vi "运维调试_氨氮.vi"() -> ()   [LabVIEW 2016, in "斯坦道氨氮.lvlib"]
uses:
  <vilib>/Utility/miscctls.llb/LVPointTypeDef.ctl
  <vilib>/Utility/config.llb/NI_LVConfig.lvlib
panel:
  in  "模块启用":bool
  in  "串口设置":bool
  in  "备用系数一键写入":bool
  in  "公式一键写入":bool
  in  "流程文件路径":path=path "C:/Users/Hsiao/Documents/斯坦道流程文件/流程.xml"
  in  "曲线模型":cluster{"X^2":dbl, "X":dbl, "B":dbl}(xcontrol)
  in  "质控参数设置":bool
  out "字符串":string
  in  "氨氮自动测试量程配置":T1
  out "ADC":sgl
  out "温度2":sgl
  out "温度1":sgl
  out "固件版本号":string
  in  "数组":string[](array[string])
  in  "备用系数写入":bool
  in  "备用系数读取":bool
  in  "备用系数":T2
  in  "量程切换阈值写入":bool
  in  "量程切换阈值读取":bool
  in  "量程切换阈值":cluster{"阈值":dbl, "标液浓度":dbl}
  in  "参数下拉列表":enum16{"氨氮", "总磷"}(ring)
  in  "量程下拉列表":enum16{"低量程", "高量程"}(ring)
  in  "测量模式下拉列表":enum16{"水样测量", "空白核查", "跨度核查", "标样核查", "加标回收"}(ring)
  in  "公式":cluster{"X^2":dbl, "X":dbl, "b":dbl}
  in  "写公式":bool
  in  "读公式":bool
  in  "返回":bool
  in  "设置":bool
  out "序列号":string="序列号"
  out "氨氮测量数据":T3(xcontrol)
  out "集成报警信息":string
  out "定时启动":bool
  out "总磷总氮运行状态":T4(xcontrol)
  in  "停止":bool
  in  "手动启动":bool
  in  "单步测试":bool
  in  "总磷氨氮调试":u16[](xcontrol)
  out "F3":sgl format="%#.6f"
  out "F2":sgl format="%#.6f"
  out "F1":sgl format="%#.6f"
  out "F0":sgl format="%#.6f"
  out "多列列表框":i32(listbox)
  # "参数设置"
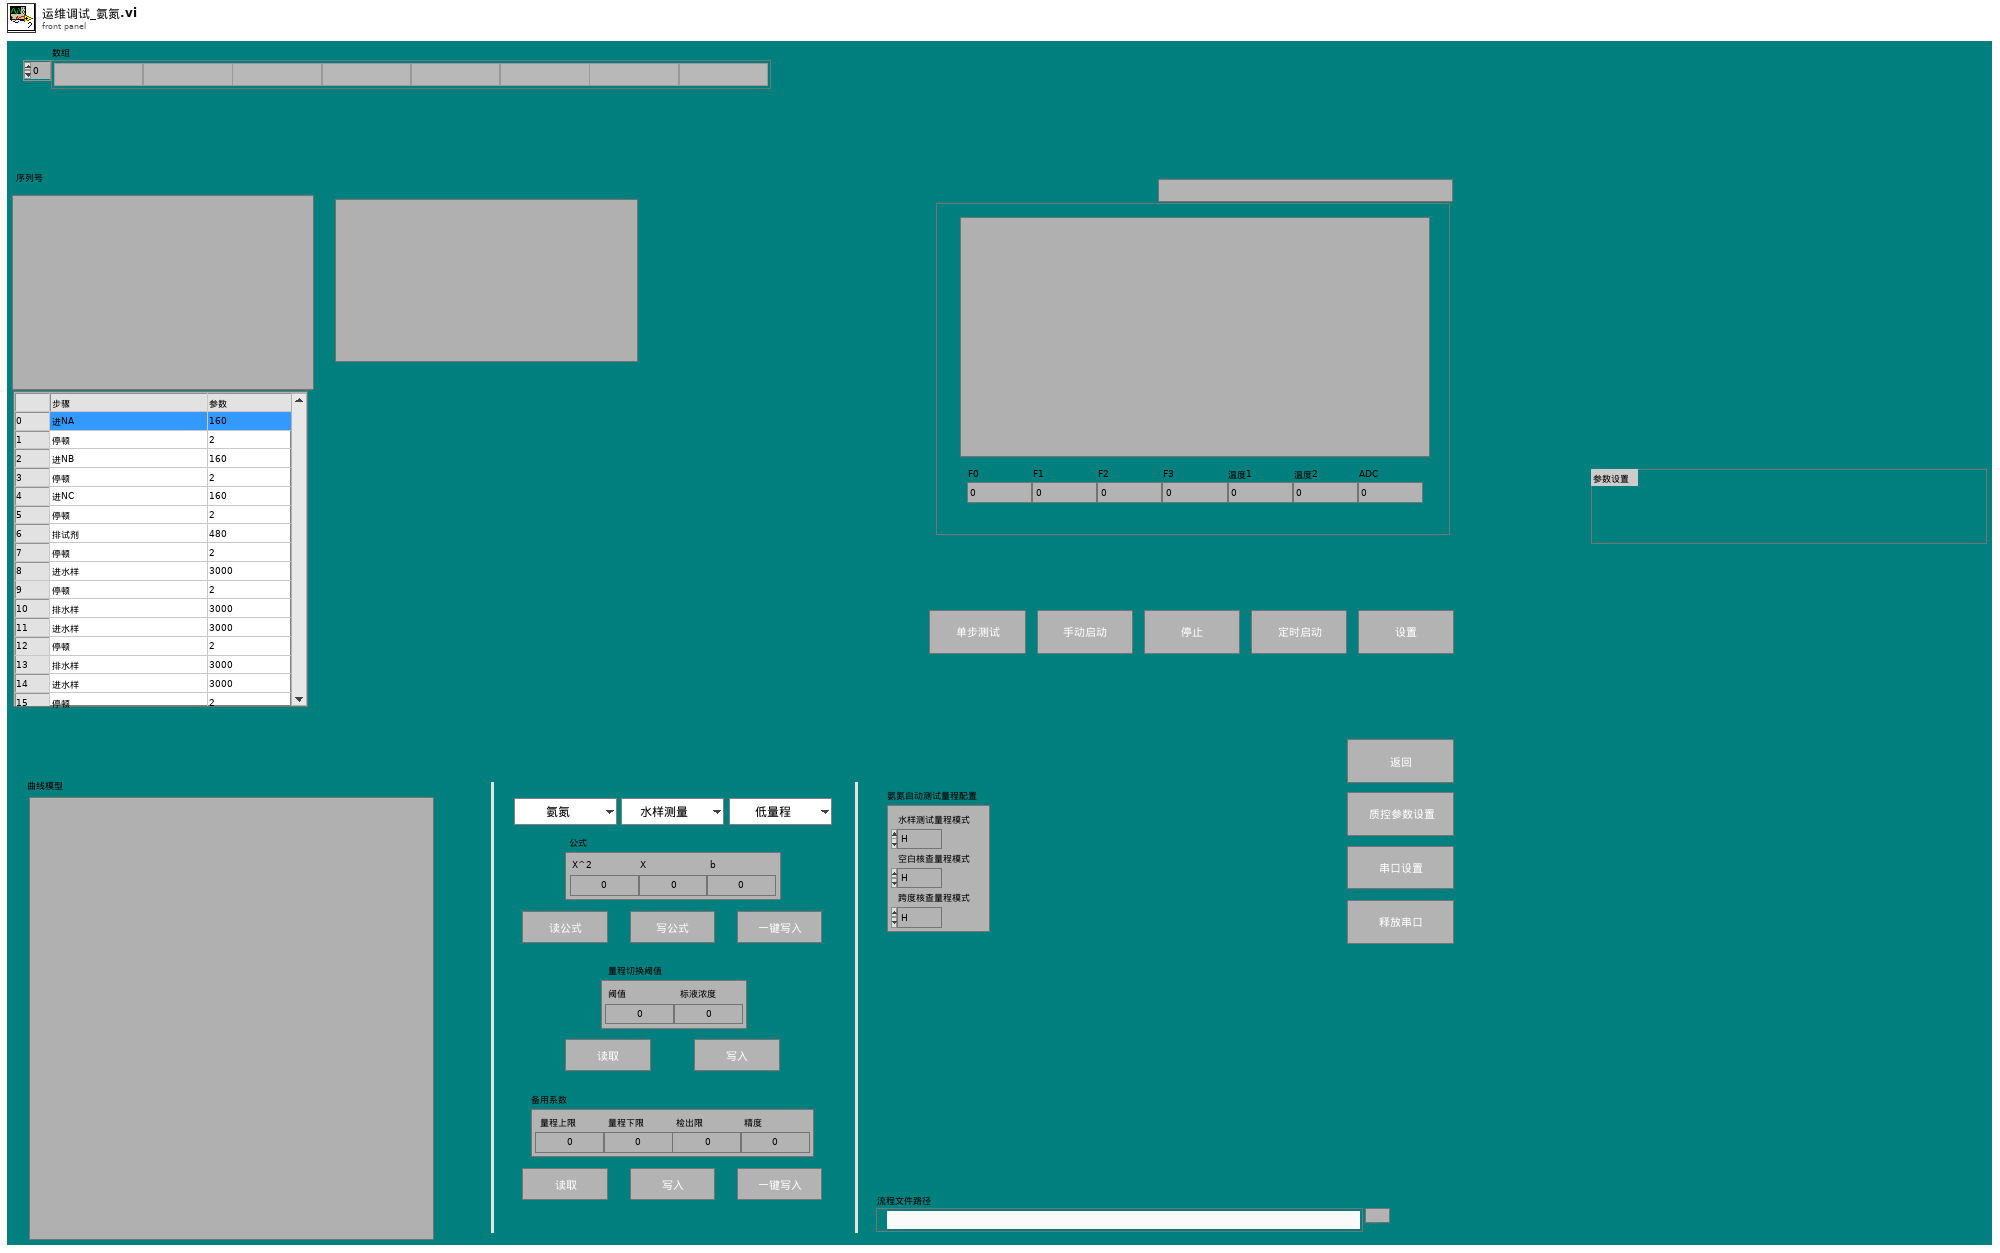
[diagram p1: front panel]
types:
  T1 = cluster{"水样测试量程模式":enum16{"H", "L", "AUTO"}, "空白核查量程模式":enum16{"H", "L", "AUTO"}, "跨度核查量程模式":enum16{"H", "L", "AUTO"}}
  T2 = cluster{"量程上限":dbl, "量程下限":dbl, "检出限":dbl, "精度":dbl}
  T3 = cluster{"flowid":u16, "测量精度":u16, "测量数据区":cluster{"因子编码":u32, "单位":u16, "标样参考值":sgl, "水样数据时间":timestamp, "水样实测值":sgl, "水样数据标识":string, "标样数据时间":timestamp, "标样实测值":sgl, "标样数据标识":string, "空白数据时间":timestamp, "空白实测值":sgl, "空白数据标识":string, "零点核查数据时间":timestamp, "零点核查实测值":sgl, "零点核查数据标识":string, "跨度核查数据时间":timestamp, "跨度核查实测值":sgl, "跨度核查数据标识":string, "加标回收数据时间":timestamp, "加标回收实测值":sgl, "加标回收数据标识":string, "平行样数据时间":timestamp, "平行样实测值":sgl, "平行样数据标识":string}}
  T4 = cluster{"系统时间":timestamp, "工作状态":enum16{"空闲", "水样测试", "标样核查", "零点核查", "跨度核查", "空白测试", "平行样测试", "加标回收", "空白校准", "标样校准", "初始化（清洗）"}, "测量模式":enum16{"待机", "连续模式", "周期模式", "定点模式", "受控模式", "手动模式"}, "告警代码":enum16{"无告警", "缺试剂告警", "缺水样告警", "缺蒸馏水告警", "缺标液告警", "仪表漏液告警", "标定异常告警", "超量程告警", "加热异常", "低试剂预警", "超上限告警", "超下限告警", "仪表内部其他异常", "滴定异常告警", "电极异常告警", "量程切换告警", "参数设置告警", "PH电极电位异常", "电导率电极异常", "浊度光度异常", "溶解氧电极异常", "溶解氧光强异常", "温度异常告警", "PH异常告警", "溶解氧异常告警", "电导率异常告警", "浊度异常告警", "叶绿素异常告警", "藻密度异常告警", "蓝绿藻异常告警", "ORP异常告警", "氨氮异常告警", "清洁刷异常告警", "SD卡异常告警", "蓝牙异常告警", "Wifi异常告警", "流程异常告警"}, "故障代码":enum16{"无故障", "电机故障", "温度故障", "通讯故障", "滴定故障"}, "日志代码":u16, "软件版本":u16, "F0":sgl, "F1":sgl, "F2":sgl, "F3":sgl, "T":sgl, "H":sgl, "id":u16, "flowid":u16, "量程":u16, "总磷控温温度1":sgl, "营养盐控温温度2":sgl, "ADC":sgl}
  T5 = cluster{"站号":u16, "量程切换":enum32{"H", "L", "AUTO"}, "控制命令":enum16{"启动测量", "标样核查", "零点核查", "跨度核查", "空白测试", "平行样测试", "加标回收", "空白校准", "标样校准", "初始化（清洗）", "停止测试", "仪器重启", "校时", "模式设置", "测量间隔设置"}, "模式设置":enum16{"待机", "连续模式", "周期模式", "定点模式", "受控模式", "手动模式"}, "测量间隔":u16}
  T6 = enum16{"启动测量", "标样核查", "零点核查", "跨度核查", "空白测试", "平行样测试", "加标回收", "空白校准", "标样校准", "初始化（清洗）", "停止测试", "仪器重启", "校时", "模式设置", "测量间隔设置"}
  T7 = cluster{"仪器测试类型":enum16{"水样测试", "标样核查", "空白测试", "跨度核查"}, "周期设置类型":enum16{"定点启动", "间隔启动"}, "定时功能启用":bool, "定时间隔":dbl, "24H周期设置":bool[]}
  T8 = enum32{"Bad", "Idle", "Run top level", "Running"}
  T9 = typedef "LVDateTimeRec.ctl" = cluster{"秒数的小数部分":dbl, "秒":i32, "分":i32, "时":i32, "日":i32, "月":i32, "年":i32, "天数（周）":i32, "天数（年）":i32, "DST":i32}
  T10 = typedef "LVPointTypeDef.ctl" = cluster{"Horizontal":i16, "Vertical":i16}
  T11 = cluster{"因子编码":u32, "单位":u16, "标样参考值":sgl, "水样数据时间":timestamp, "水样实测值":sgl, "水样数据标识":string, "标样数据时间":timestamp, "标样实测值":sgl, "标样数据标识":string, "空白数据时间":timestamp, "空白实测值":sgl, "空白数据标识":string, "零点核查数据时间":timestamp, "零点核查实测值":sgl, "零点核查数据标识":string, "跨度核查数据时间":timestamp, "跨度核查实测值":sgl, "跨度核查数据标识":string, "加标回收数据时间":timestamp, "加标回收实测值":sgl, "加标回收数据标识":string, "平行样数据时间":timestamp, "平行样实测值":sgl, "平行样数据标识":string}
  T12 = enum16{"空闲", "水样测试", "标样核查", "零点核查", "跨度核查", "空白测试", "平行样测试", "加标回收", "空白校准", "标样校准", "初始化（清洗）"}
  T13 = cluster{"启动模式":enum16{"跨度核查", "水样测量", "空白核查", "标样核查", "加标回收"}, "启动参数":u16, "量程":enum16{"低量程", "高量程"}}
  T14 = cluster{"时间标识":timestamp, "设备":string, "日志信息":string, "流程参数":string}
  T15 = cluster{"时间标识":timestamp, "设备":string, "日志信息":string}
  T16 = enum16{"无告警", "缺试剂告警", "缺水样告警", "缺蒸馏水告警", "缺标液告警", "仪表漏液告警", "标定异常告警", "超量程告警", "加热异常", "低试剂预警", "超上限告警", "超下限告警", "仪表内部其他异常", "滴定异常告警", "电极异常告警", "量程切换告警", "参数设置告警", "PH电极电位异常", "电导率电极异常", "浊度光度异常", "溶解氧电极异常", "溶解氧光强异常", "温度异常告警", "PH异常告警", "溶解氧异常告警", "电导率异常告警", "浊度异常告警", "叶绿素异常告警", "藻密度异常告警", "蓝绿藻异常告警", "ORP异常告警", "氨氮异常告警", "清洁刷异常告警", "SD卡异常告警", "蓝牙异常告警", "Wifi异常告警", "流程异常告警"}
  T17 = typedef "LVRowAndColumnUnsignedTypeDef.ctl" = cluster{"Row":u32, "Column":u32}
  T18 = typedef "NI_LVConfig.lvlib/Config Data RefNum.ctl" = refnum<k1>
  T19 = cluster{"跨度值":dbl, "零点标准液浓度":dbl, "跨度标准液浓度":dbl, "标准液标准浓度":dbl}
  T20 = cluster{"确定":bool, "跨度值":dbl, "零点标准液浓度":dbl, "跨度标准液浓度":dbl, "标准液标准浓度":dbl}
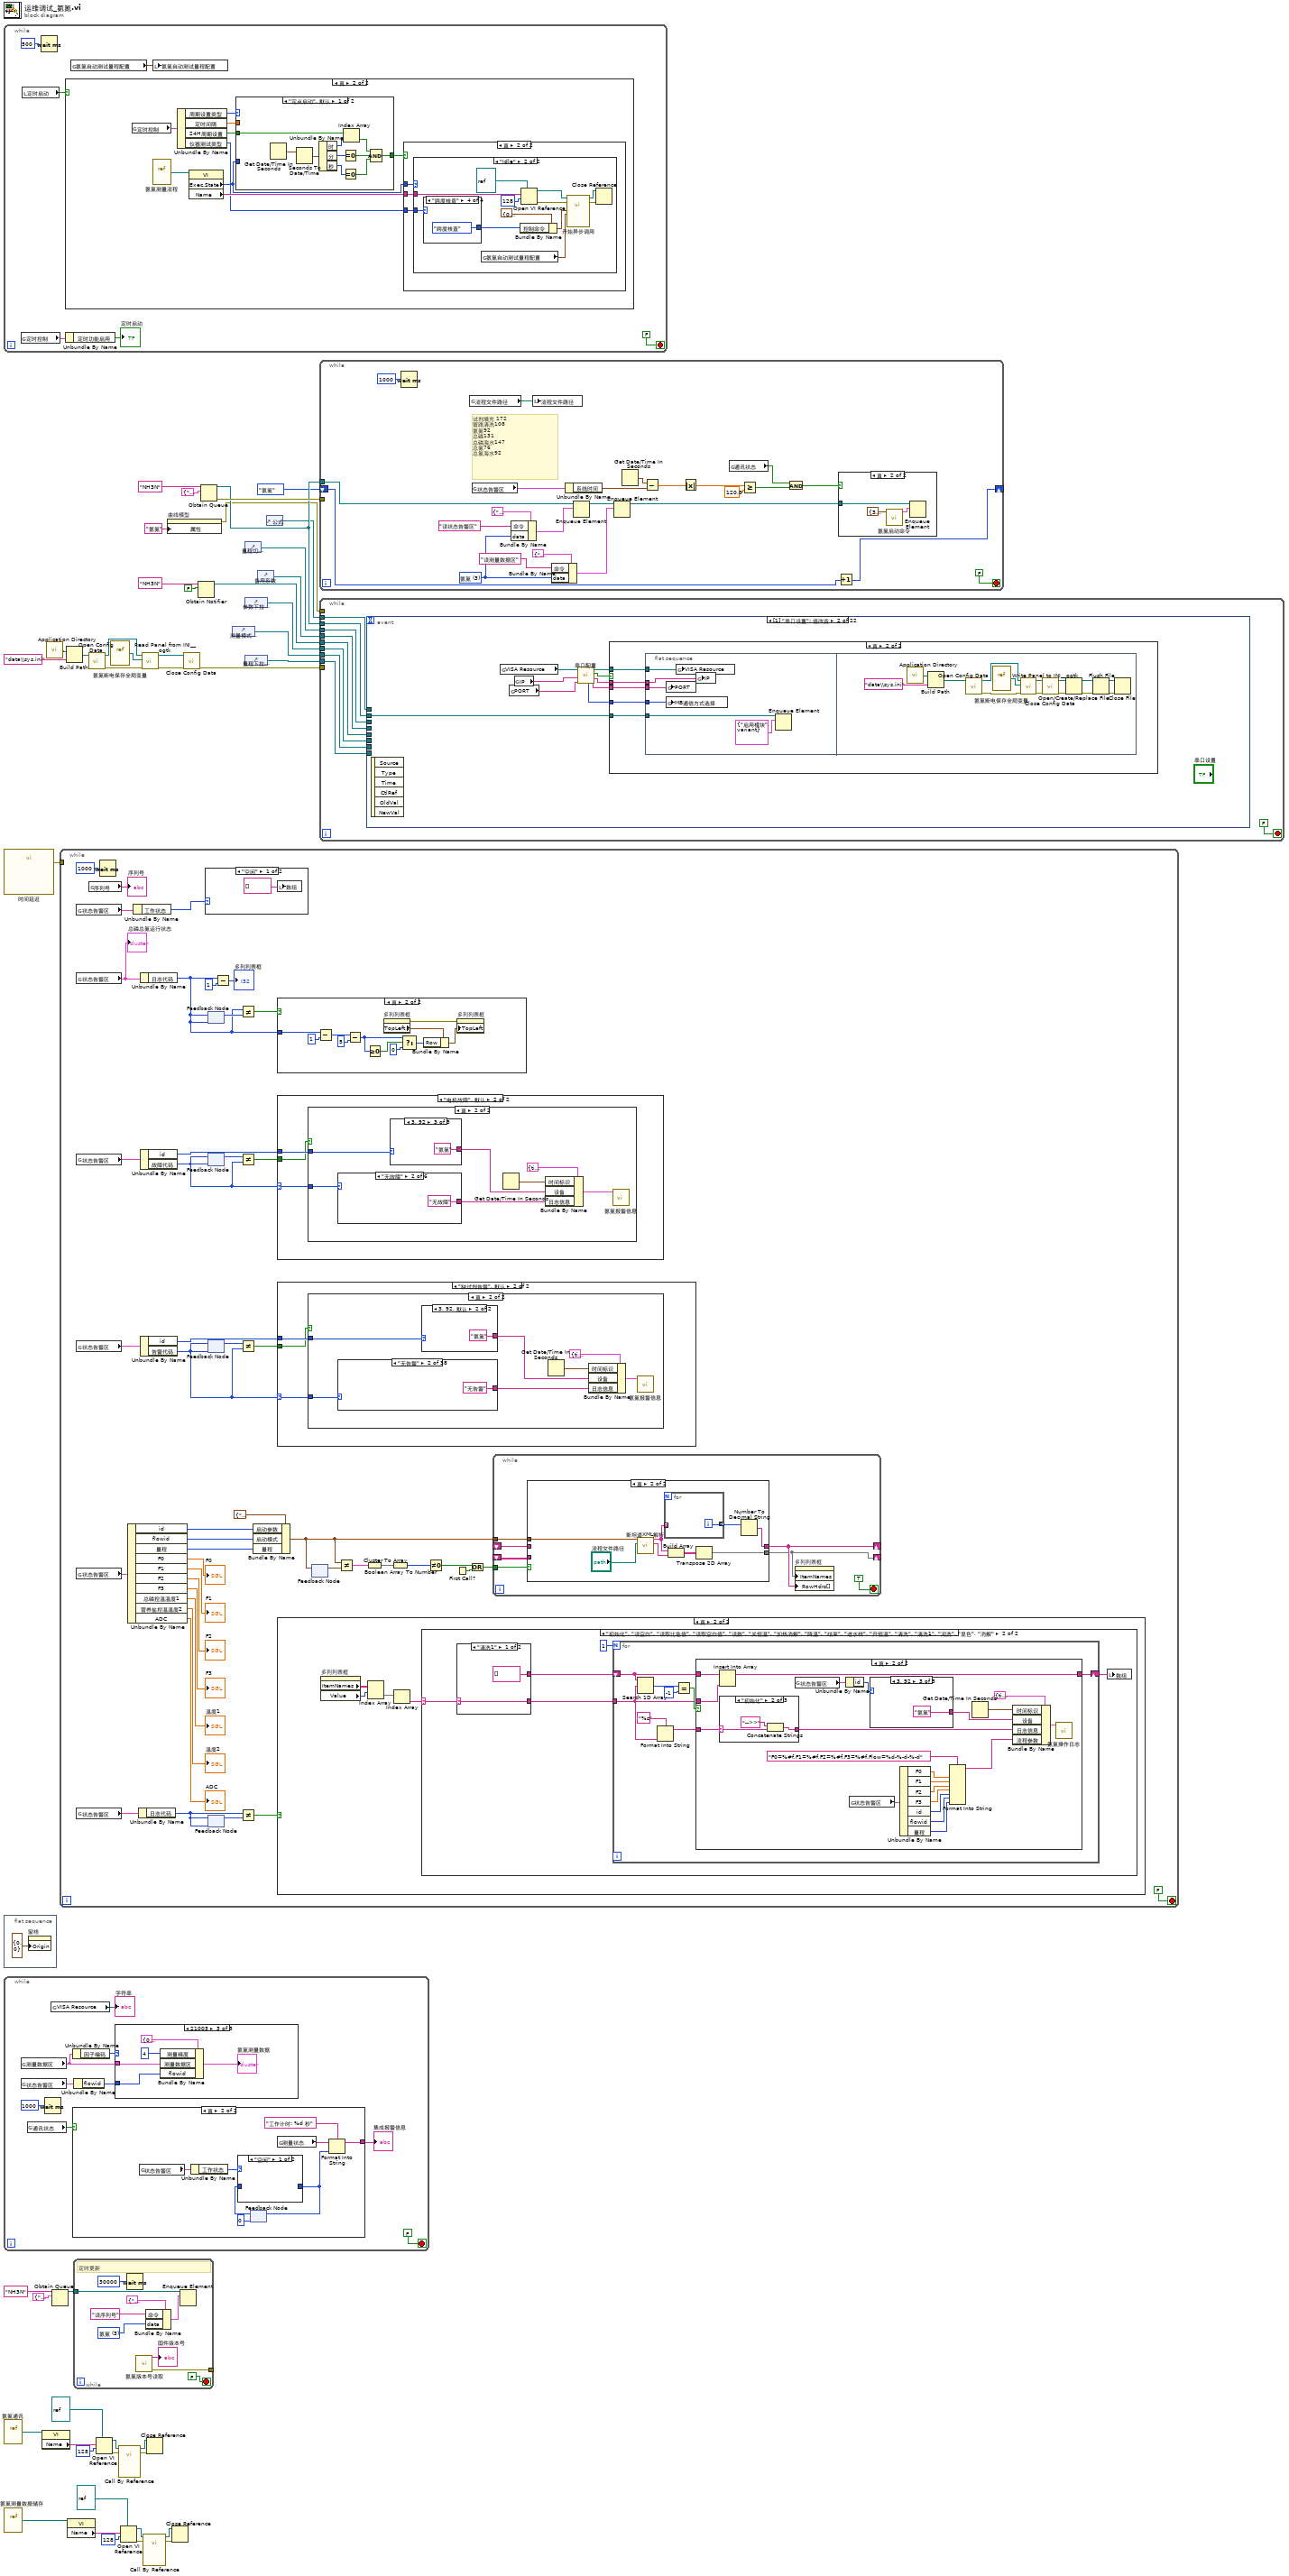
[diagram p0: block diagram]
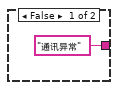
[diagram p2: hidden frame]
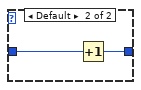
[diagram p3: hidden frame]
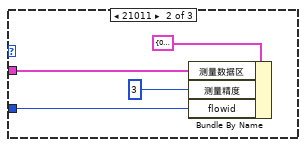
[diagram p5: hidden frame]
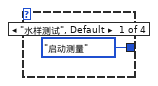
[diagram p9: hidden frame]
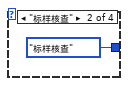
[diagram p10: hidden frame]
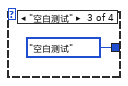
[diagram p11: hidden frame]
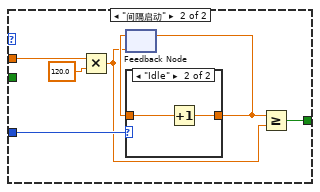
[diagram p12: hidden frame]
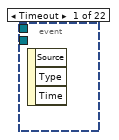
[diagram p14: hidden frame]
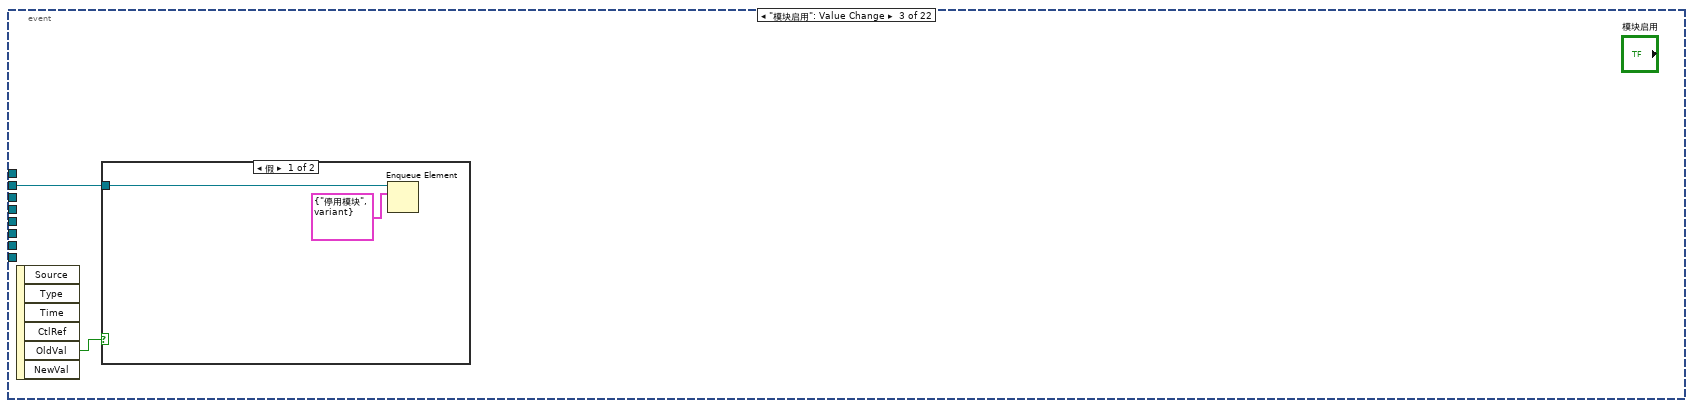
[diagram p16: hidden frame]
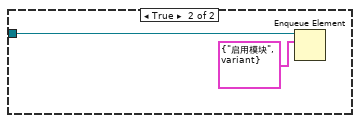
[diagram p17: hidden frame]
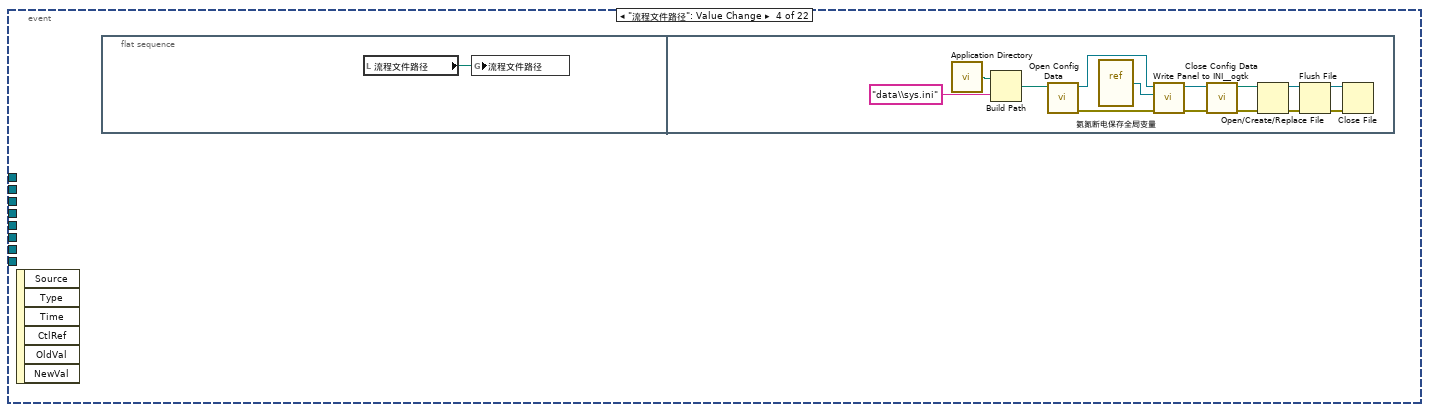
[diagram p18: hidden frame]
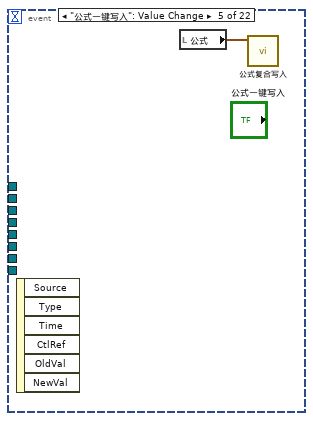
[diagram p19: hidden frame]
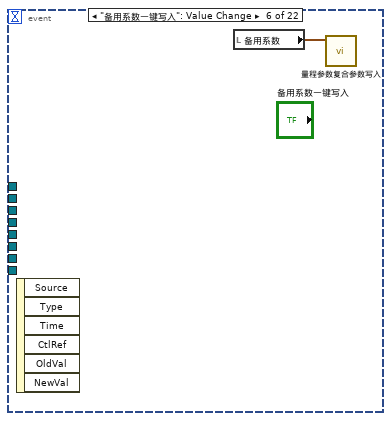
[diagram p20: hidden frame]
diagram:
  n1 = while {
    stop <- FALSE stop-if-true
    n2 = global read "氨氮断电保存全局变量.vi" "定时控制"() -> (w48:T7)
    n3 = local read "定时启动"() -> (w49:bool)
    n4 = Wait (ms)(milliseconds to wait=u32 500 ("等待时间（毫秒）")) -> ()  [unwired: 1 out]
    n5 = case shown="真" w49 {
      frame False {
      }
      frame True {
        n6 = global read "氨氮断电保存全局变量.vi" "定时控制"() -> (w60:T7)
        n7 = vi-ref "氨氮测量流程.vi"() -> (w56:refnum<vi>)
        n8 = Unbundle By Name(w60) -> ("周期设置类型"=w59:enum16{"定点启动", "间隔启动"}, "定时间隔"=w58:dbl, "24H周期设置"=w57:bool[], "仪器测试类型"=w53:enum16{"水样测试", "标样核查", "空白测试", "跨度核查"})
        n9 = property class="VI"(reference=w56) -> ("Exec.State"=w52:T8, "Name"=w55:string)  [unwired: 1 in, 2 out]
        n10 = case shown="\"定点启动\", 默认" w59 {
          tunnel: w58 -> [_ w93]
          tunnel: w57 -> [w89 _]
          tunnel: w52 -> [_ w96]
          tunnel: [w88 w91] -> w54
          frame "定点启动", Default {
            n11 = Get Date/Time In Seconds() -> (seconds since 1Jan1904=w87:timestamp)
            n12 = Seconds To Date/Time(time stamp (now)=w87) -> (date time rec=w86:T9)  [unwired: 1 in]
            n13 = Unbundle By Name(w86) -> ("时"=w85:i32, "分"=w83:i32, "秒"=w84:i32)
            n14 = Equal To 0?(x=w83) -> (x = 0?=w81:bool)
            n15 = Equal To 0?(x=w84) -> (x = 0?=w80:bool)
            n16 = Index Array(array=w89, index=w85) -> (element=w82:bool)
            n17 = Compound Arithmetic op=AND ("复合运算")(w82, w81, w80) -> (w88:bool)
          }
          frame "间隔启动" {
            n18 = Multiply(x=w93, y=120.0) -> (x*y=w90:dbl)
            n19 = feedback #1(w90) -> (w95:dbl)
            n20 = case shown="\"Idle\"" w96 {
              tunnel: w95 -> [_ w98]
              tunnel: [_ w97] -> w94
              frame "Bad", Default {
              }
              frame "Idle" {
                n21 = Increment(x=w98) -> (x+1=w97:dbl)
              }
            }
            n22 = feedback-in #1(w94) -> ()
            n23 = Greater Or Equal?(x=w94, y=w90) -> (x >= y?=w91:bool)
          }
        }
        n24 = case shown="真" w54 {
          tunnel: w55 -> [_ w63]
          tunnel: w53 -> [_ w62]
          tunnel: w52 -> [_ w61]
          frame False {
          }
          frame True {
            n25 = case shown="\"Idle\"" w61 {
              tunnel: w63 -> [_ w70]
              tunnel: w62 -> [_ w66]
              frame "Bad", Default {
              }
              frame "Idle" {
                n26 = case shown="\"跨度核查\"" w66 {
                  tunnel: [T6."启动测量" ("控制命令") T6."标样核查" ("控制命令") T6."空白测试" ("控制命令") T6."跨度核查" ("控制命令")] -> w65
                  frame "水样测试", Default {
                  }
                  frame "标样核查" {
                  }
                  frame "空白测试" {
                  }
                  frame "跨度核查" {
                  }
                }
                n27 = global read "氨氮断电保存全局变量.vi" "氨氮自动测试量程配置"() -> (w64:T1)
                n28 = Bundle By Name(cluster=T5 {"站号"=0, "量程切换"=enum."H", "控制命令"=enum."启动测量", "模式设置"=enum."待机", "测量间隔"=0} ("参数"), "控制命令"=w65) -> (w67:T5)
                n29 = Open VI Reference(type specifier VI Refnum (for type only)=refnum<vi> refnum, vi path=w70, options=128 ("选项")) -> (vi reference=w71:refnum<vi>, error out=w72:errorcluster)  [unwired: 3 in]
                n30 = call-by-ref "开始异步调用"(reference=w71, error in=w72, "量程模式"=w64, "参数"=w67) -> (reference out=w73:refnum<vi>, error out=w74:errorcluster)  [unwired: 10 in]
                n31 = Close Reference(reference=w73, error in (no error)=w74) -> ()  [unwired: 1 out]
              }
            }
          }
        }
      }
    }
    n32 = Unbundle By Name(w48) -> ("定时功能启用"=→"定时启动":bool)
    n33 = global read "氨氮断电保存全局变量.vi" "氨氮自动测试量程配置"() -> (w46:T1)
    n34 = local write "氨氮自动测试量程配置"(w46) -> ()
  }
  n35 = call "时间延迟"() -> ("error out"=w18:errorcluster)  [unwired: 11 in]
  n36 = flat-sequence {
    frame #0 {
      n37 = property on="窗格" class="Pane"("Origin"=T10 {"Horizontal"=0, "Vertical"=0} ("原点")) -> ()  [unwired: 2 in, 2 out]
    }
  }
  n38 = while {
    stop <- FALSE stop-if-true
    n39 = global read "VAR氨氮全局变量.vi" "测量数据区"() -> (w106:T11)
    n40 = global read "VAR氨氮全局变量.vi" "状态告警区"() -> (w102:T4)
    n41 = global read "VAR氨氮全局变量.vi" "通讯状态"() -> (w104:bool)
    n42 = Wait (ms)(milliseconds to wait=u32 1000 ("等待时间（毫秒）")) -> ()  [unwired: 1 out]
    n43 = global read "氨氮断电保存全局变量.vi" "VISA Resource"() -> (→"字符串":refnum<visa-resource-name>)
    n44 = Unbundle By Name(w106) -> ("因子编码"=w105:u32)
    n45 = case shown="真" w104 {
      tunnel: ["通讯异常" ("集成报警信息") w111] -> w103
      frame False {
      }
      frame True {
        n46 = global read "VAR氨氮全局变量.vi" "状态告警区"() -> (w117:T4)
        n47 = Unbundle By Name(w117) -> ("工作状态"=w116:T12)
        n48 = feedback #2(0) -> (w114:i32)
        n49 = case shown="\"空闲\"" w116 {
          tunnel: w114 -> [_ w119]
          tunnel: [_ w118] -> w112
          frame "空闲" {
          }
          frame Default {
            n50 = Increment(x=w119) -> (x+1=w118:i32)
          }
        }
        n51 = feedback-in #2(w112) -> ()
        n52 = global read "VAR氨氮全局变量.vi" "测量状态"() -> (w110:string)
        n53 = Format Into String(format string="工作计时: %d 秒" ("格式字符串"), initial string=w110, w112) -> (resulting string=w111:string)  [unwired: 1 in, 1 out]
      }
    }
    "集成报警信息" <- w103
    n54 = Unbundle By Name(w102) -> ("flowid"=w101:u16)
    n55 = case shown="21003" w105 {
      tunnel: w106 -> [_ w123 w128]
      tunnel: w101 -> [_ w121 w126]
      frame Default {
      }
      frame 21011 {
        n56 = Bundle By Name(cluster=T3 {"flowid"=0, "测量精度"=0, "测量数据区"={"因子编码"=0, "单位"=0, "标样参考值"=0.0, "水样数据时间"=timestamp(0 s since 1904-01-01), "水样实测值"=0.0, "水样数据标识"="", "标样数据时间"=timestamp(0 s since 1904-01-01), "标样实测值"=0.0, "标样数据标识"="", "空白数据时间"=timestamp(0 s since 1904-01-01), "空白实测值"=0.0, "空白数据标识"="", "零点核查数据时间"=timestamp(0 s since 1904-01-01), "零点核查实测值"=0.0, "零点核查数据标识"="", "跨度核查数据时间"=timestamp(0 s since 1904-01-01), "跨度核查实测值"=0.0, "跨度核查数据标识"="", "加标回收数据时间"=timestamp(0 s since 1904-01-01), "加标回收实测值"=0.0, "加标回收数据标识"="", "平行样数据时间"=timestamp(0 s since 1904-01-01), "平行样实测值"=0.0, "平行样数据标识"=""}} ("氨氮测量数据"), "测量数据区"=w123, "测量精度"=u16 3, "flowid"=w121) -> ()  [unwired: 1 out]
      }
      frame 21003 {
        n57 = Bundle By Name(cluster=T3 {"flowid"=0, "测量精度"=0, "测量数据区"={"因子编码"=0, "单位"=0, "标样参考值"=0.0, "水样数据时间"=timestamp(0 s since 1904-01-01), "水样实测值"=0.0, "水样数据标识"="", "标样数据时间"=timestamp(0 s since 1904-01-01), "标样实测值"=0.0, "标样数据标识"="", "空白数据时间"=timestamp(0 s since 1904-01-01), "空白实测值"=0.0, "空白数据标识"="", "零点核查数据时间"=timestamp(0 s since 1904-01-01), "零点核查实测值"=0.0, "零点核查数据标识"="", "跨度核查数据时间"=timestamp(0 s since 1904-01-01), "跨度核查实测值"=0.0, "跨度核查数据标识"="", "加标回收数据时间"=timestamp(0 s since 1904-01-01), "加标回收实测值"=0.0, "加标回收数据标识"="", "平行样数据时间"=timestamp(0 s since 1904-01-01), "平行样实测值"=0.0, "平行样数据标识"=""}} ("氨氮测量数据"), "测量精度"=u16 4, "测量数据区"=w128, "flowid"=w126) -> (→"氨氮测量数据":T3)
      }
    }
  }
  n58 = vi-ref "氨氮通讯.vi"() -> (w41:refnum<vi>)
  n59 = vi-ref "氨氮测量数据储存.vi"() -> (w33:refnum<vi>)
  n60 = property class="VI"(reference=w41) -> ("Name"=w40:string)  [unwired: 1 in, 2 out]
  n61 = call <vilib>:"Application Directory.vi"() -> ("Application Directory"=w4:path)
  n62 = Obtain Queue(name (unnamed)="NH3N" ("名称（未命名）"), element data type=cluster{"命令":string, "data":variant} {"命令"="", "data"=variant}) -> (queue out=w15:refnum<queue>)  [unwired: 3 in, 2 out]
  n63 = while {
    tunnel: w18 -> [_]
    stop <- FALSE stop-if-true
    n64 = global read "VAR氨氮全局变量.vi" "状态告警区"() -> (w141:T4)
    n65 = global read "VAR氨氮全局变量.vi" "状态告警区"() -> (w154:T4)
    "总磷总氮运行状态" <- w154
    n66 = global read "VAR氨氮全局变量.vi" "状态告警区"() -> (w146:T4)
    n67 = global read "VAR氨氮全局变量.vi" "状态告警区"() -> (w151:T4)
    n68 = global read "VAR氨氮全局变量.vi" "状态告警区"() -> (w162:T4)
    n69 = global read "VAR氨氮全局变量.vi" "状态告警区"() -> (w138:T4)
    n70 = global read "VAR氨氮全局变量.vi" "序列号"() -> (→"序列号":string)
    n71 = Wait (ms)(milliseconds to wait=u32 1000 ("等待时间（毫秒）")) -> ()  [unwired: 1 out]
    n72 = Unbundle By Name(w162) -> ("id"=w159:u16, "flowid"=w161:u16, "量程"=w160:u16, "F0"=→"F0":sgl, "F1"=→"F1":sgl, "F2"=→"F2":sgl, "F3"=→"F3":sgl, "总磷控温温度1"=→"温度1":sgl, "营养盐控温温度2"=→"温度2":sgl, "ADC"=→"ADC":sgl)
    n73 = Unbundle By Name(w141) -> ("工作状态"=w140:T12)
    n74 = Unbundle By Name(w138) -> ("日志代码"=w137:u16)
    n75 = Unbundle By Name(w154) -> ("日志代码"=w131:u16)
    n76 = Unbundle By Name(w146) -> ("id"=w145:u16, "故障代码"=w142:enum16{"无故障", "电机故障", "温度故障", "通讯故障", "滴定故障"})
    n77 = Unbundle By Name(w151) -> ("id"=w150:u16, "告警代码"=w147:T16)
    n78 = case shown="\"空闲\"" w140 {
      frame "空闲" {
        n79 = local write "数组"(string[] [] ("数组")) -> ()
      }
      frame "水样测试", Default {
      }
    }
    n80 = feedback-in #3(w131) -> ()
    n81 = feedback #3(w131) -> (w171:u16)
    n82 = feedback #4(w142) -> (w143:enum16{"无故障", "电机故障", "温度故障", "通讯故障", "滴定故障"})
    n83 = feedback-in #4(w142) -> ()
    n84 = feedback #5(w147) -> (w148:T16)
    n85 = feedback-in #5(w147) -> ()
    n86 = feedback #6(w137) -> (w139:u16)
    n87 = feedback-in #6(w137) -> ()
    n88 = Subtract(x=w131, y=1) -> (x-y=→"多列列表框":i32)
    n89 = Not Equal?(x=w131, y=w171) -> (x != y?=w170:bool)
    n90 = Not Equal?(x=w143, y=w142) -> (x != y?=w144:bool)
    n91 = Not Equal?(x=w148, y=w147) -> (x != y?=w149:bool)
    n92 = Not Equal?(x=w137, y=w139) -> (x != y?=w136:bool)
    n93 = Bundle By Name(cluster=T13 {"启动模式"=enum."跨度核查", "启动参数"=1, "量程"=enum."低量程"} ("参数簇"), "启动参数"=w159, "启动模式"=w161, "量程"=w160) -> (w153:T13)
    n94 = case shown="真" w170 {
      tunnel: w131 -> [_ w321]
      frame False {
      }
      frame True {
        n95 = Subtract(x=w321, y=1) -> (x-y=w319:i32)
        n96 = Subtract(x=w319, y=5) -> (x-y=w323:i32)
        n97 = Greater Or Equal To 0?(x=w323) -> (x >= 0?=w322:bool)
        n98 = property on="多列列表框" class="MCListbox (严格)"() -> (error out=w327:errorcluster, "TopLeft"=w328:T17)  [unwired: 2 in, 1 out]
        n99 = Select(t=w323, s=w322, f=0) -> (s? t:f=w324:i32)
        n100 = Bundle By Name(cluster=w328, "Row"=w324) -> (w329:T17)
        n101 = property on="多列列表框" class="MCListbox (严格)"(error in=w327, "TopLeft"=w329) -> ()  [unwired: 1 in, 2 out]
      }
    }
    n102 = case shown="\"电机故障\", 默认" w142 {
      selector: w142 -> [_ w228]
      tunnel: w145 -> [_ w229]
      tunnel: w144 -> [_ w227]
      frame "无故障" {
      }
      frame "电机故障", Default {
        n103 = case shown="真" w227 {
          tunnel: w229 -> [_ w236]
          tunnel: w228 -> [_ w231]
          frame False {
          }
          frame True {
            n104 = case shown="\"无故障\"" w231 {
              selector: w231 -> [w238 _ _ _ _ _]
              tunnel: [w237 "无故障" "电机故障" "温度故障" "通讯故障" "滴定故障"] -> w230
              frame Default {
                n105 = Format Into String(format string="%d" ("格式字符串"), initial string="未知" ("工作状态"), w238) -> (resulting string=w237:string)  [unwired: 1 in, 1 out]
              }
              frame "无故障" {
              }
              frame "电机故障" {
              }
              frame "温度故障" {
              }
              frame "通讯故障" {
              }
              frame "滴定故障" {
              }
            }
            n106 = case shown="3, 92" w236 {
              tunnel: [_ "总磷" ("table输入") "氨氮" ("table输入")] -> w232
              frame Default {
              }
              frame 1, 131 {
              }
              frame 3, 92 {
              }
            }
            n107 = Get Date/Time In Seconds() -> (seconds since 1Jan1904=w233:timestamp)
            n108 = Bundle By Name(cluster=T15 {"时间标识"=timestamp(0 s since 1904-01-01), "设备"="", "日志信息"=""} ("data in"), "时间标识"=w233, "设备"=w232, "日志信息"=w230) -> (w234:T15)
            n109 = call "氨氮报警信息.vi"("data in"=w234) -> ()  [unwired: 11 in]
          }
        }
      }
    }
    n110 = case shown="\"缺试剂告警\", 默认" w147 {
      selector: w147 -> [_ w249]
      tunnel: w150 -> [_ w250]
      tunnel: w149 -> [_ w248]
      frame "无告警" {
      }
      frame "缺试剂告警", Default {
        n111 = case shown="真" w248 {
          tunnel: w250 -> [_ w257]
          tunnel: w249 -> [_ w251]
          frame False {
          }
          frame True {
            n112 = case shown="\"无告警\"" w251 {
              selector: w251 -> [w259 _ _ _ _ _ _ _ _ _ _ _ _ _ _ _ _ _ _ _ _ _ _ _ _ _ _ _ _ _ _ _ _ _ _ _ _ _]
              tunnel: [w258 "无告警" "缺试剂告警" "缺水样告警" "缺蒸馏水告警" "缺标液告警" "仪表漏液告警" "标定异常告警" "超量程告警" "加热异常" "低试剂预警" "超上限告警" "超下限告警" "仪表内部其他异常" "滴定异常告警" "电极异常告警" "量程切换告警" "参数设置告警" "PH电极电位异常" "电导率电极异常" "浊度光度异常" "溶解氧电极异常" "溶解氧光强异常" "温度异常告警" "PH异常告警" "溶解氧异常告警" "电导率异常告警" "浊度异常告警" "叶绿素异常告警" "藻密度异常告警" "蓝绿藻异常告警" "ORP异常告警" "氨氮异常告警" "清洁刷异常告警" "SD卡异常告警" "蓝牙异常告警" "WiFi异常告警" "流程异常告警"] -> w252
              frame Default {
                n113 = Format Into String(format string="%d" ("格式字符串"), initial string="未知" ("工作状态"), w259) -> (resulting string=w258:string)  [unwired: 1 in, 1 out]
              }
              frame "无告警" {
              }
              frame "缺试剂告警" {
              }
              frame "缺水样告警" {
              }
              frame "缺蒸馏水告警" {
              }
              frame "缺标液告警" {
              }
              frame "仪表漏液告警" {
              }
              frame "标定异常告警" {
              }
              frame "超量程告警" {
              }
              frame "加热异常" {
              }
              frame "低试剂预警" {
              }
              frame "超上限告警" {
              }
              frame "超下限告警" {
              }
              frame "仪表内部其他异常" {
              }
              frame "滴定异常告警" {
              }
              frame "电极异常告警" {
              }
              frame "量程切换告警" {
              }
              frame "参数设置告警" {
              }
              frame "PH电极电位异常" {
              }
              frame "电导率电极异常" {
              }
              frame "浊度光度异常" {
              }
              frame "溶解氧电极异常" {
              }
              frame "溶解氧光强异常" {
              }
              frame "温度异常告警" {
              }
              frame "PH异常告警" {
              }
              frame "溶解氧异常告警" {
              }
              frame "电导率异常告警" {
              }
              frame "浊度异常告警" {
              }
              frame "叶绿素异常告警" {
              }
              frame "藻密度异常告警" {
              }
              frame "蓝绿藻异常告警" {
              }
              frame "ORP异常告警" {
              }
              frame "氨氮异常告警" {
              }
              frame "清洁刷异常告警" {
              }
              frame "SD卡异常告警" {
              }
              frame "蓝牙异常告警" {
              }
              frame "Wifi异常告警" {
              }
              frame "流程异常告警" {
              }
            }
            n114 = case shown="3, 92, 默认" w257 {
              tunnel: ["总磷" ("table输入") "氨氮" ("table输入")] -> w253
              frame 1, 131 {
              }
              frame 3, 92, Default {
              }
            }
            n115 = Get Date/Time In Seconds() -> (seconds since 1Jan1904=w254:timestamp)
            n116 = Bundle By Name(cluster=T15 {"时间标识"=timestamp(0 s since 1904-01-01), "设备"="", "日志信息"=""} ("data in"), "时间标识"=w254, "设备"=w253, "日志信息"=w252) -> (w255:T15)
            n117 = call "氨氮报警信息.vi"("data in"=w255) -> ()  [unwired: 11 in]
          }
        }
      }
    }
    n118 = case shown="真" w136 {
      frame False {
      }
      frame True {
        n119 = property on="多列列表框" class="MCListbox (严格)"() -> ("ItemNames"=w177:string[][], "Value"=w178:i32)  [unwired: 2 in, 2 out]
        n120 = Index Array(array=w177, index (row)=w178) -> (element=w176:string[])  [unwired: 1 in]
        n121 = Index Array(array=w176) -> (element=w175:string)  [unwired: 1 in]
        n122 = case shown="\"初始化\", \"读空白\", \"读取比色值\", \"读取空白值\", \"读数\", \"关恒温\", \"加热消解\", \"降温\", \"结束\", \"进水样\", \"开恒温\", \"清洗\", \"清洗1\", \"润洗\", \"显色\", \"消解\"" w175 {
          selector: w175 -> [_ w181]
          frame Default {
          }
          frame "初始化", "读空白", "读取比色值", "读取空白值", "读数", "关恒温", "加热消解", "降温", "结束", "进水样", "开恒温", "清洗", "清洗1", "润洗", "显色", "消解" {
            n123 = case shown="\"清洗1\"" w181 {
              selector: w181 -> [w185 w187]
              tunnel: [w185 w187] -> w180
              tunnel: [string[] [] ("数组") "数组"] -> w179
              frame "清洗1" {
              }
              frame Default {
              }
            }
            n124 = for {
              N: 1 -> [_]
              tunnel: w180 -> [w189]
              shift-right: [w188] -> w182
              shift-left: w179 -> [w190]
              n125 = Search 1D Array(1D array=w190, element=w189) -> (index of element=w193:i32)  [unwired: 1 in]
              n126 = Format Into String(format string="%s" ("格式字符串"), w189) -> (resulting string=w194:string)  [unwired: 2 in, 1 out]
              n127 = Equal?(x=w193, y=-1) -> (x = y?=w191:bool)
              n128 = case shown="真" w191 {
                tunnel: w194 -> [_ w198]
                tunnel: w190 -> [w196 w202]
                tunnel: w189 -> [_ w201]
                tunnel: [w196 w200] -> w188
                frame False {
                }
                frame True {
                  n129 = Insert Into Array(array=w202, new element=w201) -> (w200:string[])  [unwired: 1 in]
                  n130 = case shown="\"初始化\"" w198 {
                    selector: w198 -> [w218 w221 w224]
                    tunnel: [w218 w220 w223] -> w197
                    frame Default {
                    }
                    frame "初始化" {
                      n131 = Concatenate Strings("-->>" ("字符串"), w221) -> (w220:string)
                    }
                    frame "结束" {
                      n132 = Concatenate Strings("-->>" ("字符串"), w224) -> (w223:string)
                    }
                  }
                  n133 = global read "VAR氨氮全局变量.vi" "状态告警区"() -> (w217:T4)
                  n134 = Unbundle By Name(w217) -> ("id"=w216:u16)
                  n135 = global read "VAR氨氮全局变量.vi" "状态告警区"() -> (w212:T4)
                  n136 = case shown="3, 92" w216 {
                    tunnel: [_ "总磷" ("table输入") "氨氮" ("table输入")] -> w214
                    frame Default {
                    }
                    frame 1, 131 {
                    }
                    frame 3, 92 {
                    }
                  }
                  n137 = Unbundle By Name(w212) -> ("F0"=w209:sgl, "F1"=w208:sgl, "F2"=w207:sgl, "F3"=w206:sgl, "id"=w205:u16, "flowid"=w204:u16, "量程"=w203:u16)
                  n138 = Format Into String(format string="F0=%#f,F1=%#f,F2=%#f,F3=%#f,Flow=%d-%-d-%-d" ("格式字符串"), w209, w208, w207, w206, w205, w204, w203) -> (resulting string=w210:string)  [unwired: 2 in, 1 out]
                  n139 = Get Date/Time In Seconds() -> (seconds since 1Jan1904=w213:timestamp)
                  n140 = Bundle By Name(cluster=T14 {"时间标识"=timestamp(0 s since 1904-01-01), "设备"="", "日志信息"="", "流程参数"=""} ("data in"), "时间标识"=w213, "设备"=w214, "日志信息"=w197, "流程参数"=w210) -> (w215:T14)
                  n141 = call "氨氮操作日志.vi"("data in"=w215) -> ()  [unwired: 11 in]
                }
              }
            }
            n142 = local write "数组"(w182) -> ()
          }
        }
      }
    }
    n143 = feedback #7() -> (w166:T13)  [unwired: 1 in]
    n144 = feedback-in #7(w153) -> ()
    n145 = Not Equal?(x=w153, y=w166) -> (x != y?=w167:cluster{"启动模式":bool, "启动参数":bool, "量程":bool})
    n146 = Cluster To Array(cluster=w167) -> (array=w168:bool[])
    n147 = Boolean Array To Number(Boolean array=w168) -> (number=w169:u32)
    n148 = Not Equal To 0?(x=w169) -> (x != 0?=w164:bool)
    n149 = First Call?() -> (First Call?: T/F=w165:bool)
    n150 = Or(x=w164, y=w165) -> (x .or. y?=w163:bool)
    n151 = while {
      tunnel: w163 -> [w307]
      tunnel: w153 -> [w306]
      shift-right: [w301] -> _
      shift-left: _ -> [w303]
      shift-right: [w302] -> _
      shift-left: _ -> [w304]
      stop <- TRUE stop-if-true
      n152 = case shown="真" w307 {
        tunnel: [w309 w317] -> w302
        tunnel: [w308 w316] -> w301
        tunnel: w306 -> [_ w311]
        tunnel: w304 -> [w309 _]
        tunnel: w303 -> [w308 _]
        frame False {
        }
        frame True {
          n153 = call "斯坦道XML解析.vi"("添加的路径"="流程文件路径", "参数簇"=w311) -> ("步骤时间"=w312:string[], "步骤名"=w314:string[])  [unwired: 8 in]
          n154 = for {
            tunnel: w314 -> [_] mode=indexing
            tunnel: [w318] -> w315 mode=indexing
            i -> [w318]
          }
          n155 = Build Array(w314, w312) -> (w313:string[][])
          n156 = Transpose 2D Array(2D array=w313) -> (transposed array=w316:string[][])
          n157 = Number To Decimal String(number=w315) -> (decimal integer string=w317:string[])  [unwired: 1 in]
        }
      }
      n158 = property on="多列列表框" class="MCListbox (严格)"("ItemNames"=w301, "RowHdrs[]"=w302) -> ()  [unwired: 2 in, 2 out]
    }
  }
  n159 = Build Path(base path=w4, name or relative path="data\\sys.ini" ("名称或相对路径")) -> (appended path=w6:path)
  n160 = property class="VI"(reference=w33) -> ("Name"=w26:string)  [unwired: 1 in, 2 out]
  n161 = while {
    tunnel: w15 -> [w334]
    tunnel: [w331] -> _
    stop <- FALSE stop-if-true
    w335 = u16 3 items=["总磷"=1, "氨氮"=3] ("站号")
    # "定时更新"
    n162 = Wait (ms)(milliseconds to wait=u32 30000 ("等待时间（毫秒）")) -> ()  [unwired: 1 out]
    n163 = call "氨氮版本号读取.vi"() -> ("error out"=w331:errorcluster, "固件版本号"=→"固件版本号":string)  [unwired: 10 in]
    n164 = Bundle By Name(cluster=cluster{"命令":string, "data":variant} {"命令"="", "data"=variant} ("元素"), "命令"="读序列号", "data"=w335) -> (w333:cluster{"命令":string, "data":variant})
    n165 = Enqueue Element(queue=w334, element=w333) -> ()  [unwired: 2 in, 3 out]
  }
  n166 = call <vilib>:"Open Config Data.vi"("configuration file path"=w6) -> ("error out"=w10:errorcluster, "refnum"=w7:T18)  [unwired: 8 in, 1 out]
  n167 = Open VI Reference(type specifier VI Refnum (for type only)=refnum<vi> refnum, vi path=w40, options=128 ("选项")) -> (vi reference=w38:refnum<vi>, error out=w36:errorcluster)  [unwired: 3 in]
  n168 = vi-ref "氨氮断电保存全局变量.vi"() -> (w8:refnum<vi>)
  n169 = call-by-ref "?"(reference=w38, error in=w36) -> (reference out=w34:refnum<vi>, error out=w35:errorcluster)  [unwired: 12 in]
  n170 = Open VI Reference(type specifier VI Refnum (for type only)=refnum<vi> refnum, vi path=w26, options=128 ("选项")) -> (vi reference=w28:refnum<vi>, error out=w30:errorcluster)  [unwired: 3 in]
  n171 = call <userlib>:"Read Panel from INI__ogtk.vi"("error in (no error)"=w10, "VI ref"=w8, "refnum"=w7) -> ("error out"=w11:errorcluster, "refnum out"=w9:T18)  [unwired: 7 in]
  n172 = call-by-ref "?"(reference=w28, error in=w30) -> (reference out=w32:refnum<vi>, error out=w31:errorcluster)  [unwired: 12 in]
  n173 = Close Reference(reference=w34, error in (no error)=w35) -> ()  [unwired: 1 out]
  n174 = property on="曲线模型" class="氨氮曲线模型 (严格)"("属性"="氨氮" ("调用模块名称属性")) -> (error out=w2:errorcluster)  [unwired: 2 in, 1 out]
  n175 = Close Reference(reference=w32, error in (no error)=w31) -> ()  [unwired: 1 out]
  n176 = call <vilib>:"Close Config Data.vi"("error in (no error)"=w11, "refnum"=w9) -> ("error out"=w3:errorcluster)  [unwired: 8 in, 1 out]
  n177 = Obtain Notifier(name (unnamed)="NH3N" ("名称（未命名）"), notification data type=FALSE) -> (notifier out=w12:refnum<notifier>)  [unwired: 2 in, 2 out]
  n178 = Obtain Queue(name (unnamed)="NH3N" ("名称（未命名）"), element data type=cluster{"命令":string, "data":variant} {"命令"="", "data"=variant}) -> (queue out=w42:refnum<queue>, error out=w43:errorcluster)  [unwired: 3 in, 1 out]
  n179 = control-ref of="测量模式下拉列表"() -> (w22:refnum<vi>)
  n180 = control-ref of="量程切换阈值"() -> (w20:refnum<vi>)
  n181 = control-ref of="参数下拉列表"() -> (w23:refnum<vi>)
  n182 = control-ref of="量程下拉列表"() -> (w24:refnum<vi>)
  n183 = control-ref of="备用系数"() -> (w19:refnum<vi>)
  n184 = control-ref of="公式"() -> (w21:refnum<vi>)
  n185 = while {
    tunnel: w42 -> [w357]
    tunnel: w43 -> [_]
    shift-right: [w351] -> _
    shift-left: enum16{"氨氮", "总磷"}."氨氮" ("枚举") -> [w352]
    stop <- FALSE stop-if-true
    w350 = u16 3 items=["总磷"=1, "氨氮"=3] ("站号")
    # "试剂填充 172 \n管路清洗108\n氨氮92\n总磷131\n总磷海水147\n总氮76\n总氮海水92"
    n186 = Wait (ms)(milliseconds to wait=u32 1000 ("等待时间（毫秒）")) -> ()  [unwired: 1 out]
    n187 = global read "氨氮断电保存全局变量.vi" "流程文件路径"() -> (w339:path)
    n188 = global read "VAR氨氮全局变量.vi" "状态告警区"() -> (w348:T4)
    n189 = Bundle By Name(cluster=cluster{"命令":string, "data":variant} {"命令"="", "data"=variant} ("元素"), "命令"="读状态告警区", "data"=w350) -> (w359:cluster{"命令":string, "data":variant})
    n190 = local write "流程文件路径"(w339) -> ()
    n191 = Bundle By Name(cluster=cluster{"命令":string, "data":variant} {"命令"="", "data"=variant} ("元素"), "命令"="读测量数据区", "data"=w350) -> (w355:cluster{"命令":string, "data":variant})
    n192 = Unbundle By Name(w348) -> ("系统时间"=w347:timestamp)
    n193 = Enqueue Element(queue=w357, element=w359) -> (queue out=w353:refnum<queue>)  [unwired: 2 in, 2 out]
    n194 = Enqueue Element(queue=w353, element=w355) -> (queue out=w349:refnum<queue>)  [unwired: 2 in, 2 out]
    n195 = Get Date/Time In Seconds() -> (seconds since 1Jan1904=w346:timestamp)
    n196 = Subtract(x=w346, y=w347) -> (x-y=w345:dbl)
    n197 = Absolute Value(x=w345) -> (abs(x)=w344:dbl)
    n198 = global read "VAR氨氮全局变量.vi" "通讯状态"() -> (w340:bool)
    n199 = Greater Or Equal?(x=w344, y=120.0) -> (x >= y?=w342:bool)
    n200 = And(x=w340, y=w342) -> (x .and. y?=w341:bool)
    n201 = case shown="真" w341 {
      tunnel: w349 -> [_ w364]
      frame False {
      }
      frame True {
        n202 = call "氨氮启动命令.vi"("参数"=T5 {"站号"=3, "量程切换"=enum."AUTO", "控制命令"=enum."校时", "模式设置"=enum."待机", "测量间隔"=0}) -> ("启动命令"=w363:cluster{"命令":string, "data":variant})  [unwired: 10 in]
        n203 = Enqueue Element(queue=w364, element=w363) -> ()  [unwired: 2 in, 3 out]
      }
    }
    n204 = Increment(x=w352) -> (x+1=w351:enum16{"氨氮", "总磷"})
  }
  n205 = while {
    tunnel: w42 -> [w373]
    tunnel: w24 -> [w372]
    tunnel: w23 -> [w371]
    tunnel: w22 -> [w370]
    tunnel: w21 -> [w369]
    tunnel: w20 -> [w368]
    tunnel: w19 -> [w367]
    tunnel: w12 -> [w366]
    tunnel: w3 -> [_]
    tunnel: w2 -> [_]
    stop <- FALSE stop-if-true
    n206 = event shown="[1] \"串口设置\": 值改变" {
      selector: _ -> [_ _ _ _ _ _ _ _ _ _ _ _ _ _ _ _ _ _ _ _ _ _]
      dyn-events: _ -> [_ _ _ _ _ _ _ _ _ _ _ _ _ _ _ _ _ _ _ _ _ _]
      timeout: _ -> [_ _ _ _ _ _ _ _ _ _ _ _ _ _ _ _ _ _ _ _ _ _]
      tunnel: w373 -> [_ w380 w409 _ _ _ _ _ _ w476 _ w501 w506 _ _ _ _ _ _ _ _ _]
      tunnel: w372 -> [_ _ _ _ _ _ _ _ _ _ _ _ _ _ _ _ w522 _ w542 w551 w558 w569]
      tunnel: w371 -> [_ _ _ _ _ _ _ _ _ _ _ _ _ _ _ _ w520 _ w540 w553 w565 w576]
      tunnel: w370 -> [_ _ _ _ _ _ _ _ _ _ _ _ _ _ _ _ w521 _ w541 w552 w559 w571]
      tunnel: w369 -> [_ _ _ _ _ _ _ _ _ _ _ _ _ _ _ _ w516 _ _ _ _ _]
      tunnel: w368 -> [_ _ _ _ _ _ _ _ _ _ _ _ _ _ _ _ _ _ w536 _ _ _]
      tunnel: w367 -> [_ _ _ _ _ _ _ _ _ _ _ _ _ _ _ _ _ _ _ _ w563 _]
      tunnel: w366 -> [_ _ _ _ _ _ _ _ _ _ _ _ w504 _ _ _ _ _ _ _ _ _]
      event Timeout {
        n207 = event-data() -> ()  [unwired: 1 in, 3 out]
      }
      event "串口设置": Value Change {
        n208 = event-data() -> ()  [unwired: 1 in, 6 out]
        n209 = global read "氨氮断电保存全局变量.vi" "VISA Resource"() -> (w383:refnum<visa-resource-name>)
        n210 = global read "氨氮断电保存全局变量.vi" "PORT"() -> (w378:string)
        n211 = global read "氨氮断电保存全局变量.vi" "IP"() -> (w379:string)
        n212 = call "串口配置.vi"("PORT"=w378, "IP"=w379, "请选择串口:"=w383) -> ("PORT 2"=w376:string, "IP 2"=w377:string, "确认 2"=w382:bool, "VISA资源名称 2"=w381:refnum<visa-resource-name>, "MB通信方式选择 2"=w375:enum16{"串口", "TCP"})  [unwired: 4 in]
        n213 = case shown="真" w382 {
          tunnel: w381 -> [_ w388]
          tunnel: w380 -> [_ w387]
          tunnel: w377 -> [_ w386]
          tunnel: w376 -> [_ w385]
          tunnel: w375 -> [_ w384]
          frame False {
          }
          frame True {
            n214 = flat-sequence {
              tunnel: w388 -> [w394]
              tunnel: w387 -> [w392]
              tunnel: w386 -> [w391]
              tunnel: w385 -> [w390]
              tunnel: w384 -> [w389]
              frame #0 {
                n215 = global write "氨氮断电保存全局变量.vi" "PORT"(w390) -> ()
                n216 = global write "氨氮断电保存全局变量.vi" "MB通信方式选择"(w389) -> ()
                n217 = global write "氨氮断电保存全局变量.vi" "VISA Resource"(w394) -> ()
                n218 = global write "氨氮断电保存全局变量.vi" "IP"(w391) -> ()
                n219 = Enqueue Element(queue=w392, element=cluster{"命令":string, "data":variant} {"命令"="启用模块", "data"=variant} ("元素")) -> ()  [unwired: 2 in, 3 out]
              }
              frame #1 {
                n220 = call <vilib>:"Application Directory.vi"() -> ("Application Directory"=w408:path)
                n221 = Build Path(base path=w408, name or relative path="data\\sys.ini" ("名称或相对路径")) -> (appended path=w406:path)
                n222 = call <vilib>:"Open Config Data.vi"("configuration file path"=w406) -> ("error out"=w402:errorcluster, "refnum"=w405:T18)  [unwired: 8 in, 1 out]
                n223 = vi-ref "氨氮断电保存全局变量.vi"() -> (w404:refnum<vi>)
                n224 = call <userlib>:"Write Panel to INI__ogtk.vi"("error in (no error)"=w402, "VI ref"=w404, "refnum"=w405) -> ("error out"=w401:errorcluster, "refnum out"=w403:T18)  [unwired: 7 in]
                n225 = call <vilib>:"Close Config Data.vi"("error in (no error)"=w401, "refnum"=w403) -> ("error out"=w396:errorcluster, "file path"=w395:path)  [unwired: 8 in]
                n226 = Open/Create/Replace File(file path (use dialog)=w395, error in=w396) -> (refnum out=w399:refnum<file>, error out=w400:errorcluster)  [unwired: 4 in, 1 out]
                n227 = Flush File(refnum=w399, error in=w400) -> (refnum out=w398:refnum<file>, error out=w397:errorcluster)
                n228 = Close File(refnum=w398, error in=w397) -> ()  [unwired: 2 out]
              }
            }
          }
        }
      }
      event "模块启用": Value Change {
        n229 = event-data() -> ("OldVal"=w410:bool)  [unwired: 1 in, 5 out]
        n230 = case shown="假" w410 {
          tunnel: w409 -> [w411 w413]
          frame False {
            n231 = Enqueue Element(queue=w411, element=cluster{"命令":string, "data":variant} {"命令"="停用模块", "data"=variant} ("元素")) -> ()  [unwired: 2 in, 3 out]
          }
          frame True {
            n232 = Enqueue Element(queue=w413, element=cluster{"命令":string, "data":variant} {"命令"="启用模块", "data"=variant} ("元素")) -> ()  [unwired: 2 in, 3 out]
          }
        }
      }
      event "流程文件路径": Value Change {
        n233 = event-data() -> ()  [unwired: 1 in, 6 out]
        n234 = flat-sequence {
          frame #0 {
            n235 = local read "流程文件路径"() -> (w415:path)
            n236 = global write "氨氮断电保存全局变量.vi" "流程文件路径"(w415) -> ()
          }
          frame #1 {
            n237 = call <vilib>:"Application Directory.vi"() -> ("Application Directory"=w429:path)
            n238 = Build Path(base path=w429, name or relative path="data\\sys.ini" ("名称或相对路径")) -> (appended path=w427:path)
            n239 = call <vilib>:"Open Config Data.vi"("configuration file path"=w427) -> ("error out"=w423:errorcluster, "refnum"=w426:T18)  [unwired: 8 in, 1 out]
            n240 = vi-ref "氨氮断电保存全局变量.vi"() -> (w425:refnum<vi>)
            n241 = call <userlib>:"Write Panel to INI__ogtk.vi"("error in (no error)"=w423, "VI ref"=w425, "refnum"=w426) -> ("error out"=w422:errorcluster, "refnum out"=w424:T18)  [unwired: 7 in]
            n242 = call <vilib>:"Close Config Data.vi"("error in (no error)"=w422, "refnum"=w424) -> ("error out"=w417:errorcluster, "file path"=w416:path)  [unwired: 8 in]
            n243 = Open/Create/Replace File(file path (use dialog)=w416, error in=w417) -> (refnum out=w420:refnum<file>, error out=w421:errorcluster)  [unwired: 4 in, 1 out]
            n244 = Flush File(refnum=w420, error in=w421) -> (refnum out=w419:refnum<file>, error out=w418:errorcluster)
            n245 = Close File(refnum=w419, error in=w418) -> ()  [unwired: 2 out]
          }
        }
      }
      event "公式一键写入": Value Change {
        n246 = event-data() -> ()  [unwired: 1 in, 6 out]
        n247 = local read "公式"() -> (w430:cluster{"X^2":dbl, "X":dbl, "b":dbl})
        n248 = call "公式复合写入.vi"("公式"=w430) -> ()  [unwired: 11 in]
      }
      event "备用系数一键写入": Value Change {
        n249 = event-data() -> ()  [unwired: 1 in, 6 out]
        n250 = local read "备用系数"() -> (w431:T2)
        n251 = call "量程参数复合参数写入.vi"("备用系数"=w431) -> ()  [unwired: 11 in]
      }
      event "曲线模型": Value Change {
        n252 = event-data() -> ()  [unwired: 1 in, 6 out]
        n253 = local write "公式"("曲线模型") -> ()
      }
      event "质控参数设置": Value Change {
        n254 = event-data() -> ()  [unwired: 1 in, 6 out]
        n255 = global read "氨氮断电保存全局变量.vi" "质控参数设置"() -> (w433:T19)
        n256 = call "质控参数设置.vi"("质控参数设置"=w433) -> ("输出簇"=w434:T20)  [unwired: 10 in]
        n257 = Unbundle By Name(w434) -> ("确定"=w435:bool)
        n258 = case shown="真" w435 {
          tunnel: w434 -> [_ w437]
          tunnel: w433 -> [_ w436]
          frame False {
          }
          frame True {
            n259 = flat-sequence {
              tunnel: w437 -> [w444]
              tunnel: w436 -> [w438]
              frame #0 {
                n260 = Unbundle By Name(w444) -> ("跨度值"=w443:dbl, "零点标准液浓度"=w442:dbl, "跨度标准液浓度"=w441:dbl, "标准液标准浓度"=w440:dbl)
                n261 = Bundle By Name(cluster=w438, "跨度值"=w443, "零点标准液浓度"=w442, "跨度标准液浓度"=w441, "标准液标准浓度"=w440) -> (w439:T19)
                n262 = global write "氨氮断电保存全局变量.vi" "质控参数设置"(w439) -> ()
              }
              frame #1 {
                n263 = call <vilib>:"Application Directory.vi"() -> ("Application Directory"=w445:path)
                n264 = Build Path(base path=w445, name or relative path="data\\sys.ini" ("名称或相对路径")) -> (appended path=w447:path)
                n265 = call <vilib>:"Open Config Data.vi"("configuration file path"=w447) -> ("error out"=w451:errorcluster, "refnum"=w448:T18)  [unwired: 8 in, 1 out]
                n266 = vi-ref "氨氮断电保存全局变量.vi"() -> (w449:refnum<vi>)
                n267 = call <userlib>:"Write Panel to INI__ogtk.vi"("error in (no error)"=w451, "VI ref"=w449, "refnum"=w448) -> ("error out"=w452:errorcluster, "refnum out"=w450:T18)  [unwired: 7 in]
                n268 = call <vilib>:"Close Config Data.vi"("error in (no error)"=w452, "refnum"=w450) -> ("error out"=w457:errorcluster, "file path"=w458:path)  [unwired: 8 in]
                n269 = Open/Create/Replace File(file path (use dialog)=w458, error in=w457) -> (refnum out=w454:refnum<file>, error out=w453:errorcluster)  [unwired: 4 in, 1 out]
                n270 = Flush File(refnum=w454, error in=w453) -> (refnum out=w455:refnum<file>, error out=w456:errorcluster)
                n271 = Close File(refnum=w455, error in=w456) -> ()  [unwired: 2 out]
              }
            }
          }
        }
      }
      event "氨氮自动测试量程配置": Value Change {
        n272 = event-data() -> ()  [unwired: 1 in, 6 out]
        n273 = flat-sequence {
          frame #0 {
            n274 = global write "氨氮断电保存全局变量.vi" "氨氮自动测试量程配置"("氨氮自动测试量程配置") -> ()
          }
          frame #1 {
            n275 = call <vilib>:"Application Directory.vi"() -> ("Application Directory"=w473:path)
            n276 = Build Path(base path=w473, name or relative path="data\\sys.ini" ("名称或相对路径")) -> (appended path=w471:path)
            n277 = call <vilib>:"Open Config Data.vi"("configuration file path"=w471) -> ("error out"=w467:errorcluster, "refnum"=w470:T18)  [unwired: 8 in, 1 out]
            n278 = vi-ref "氨氮断电保存全局变量.vi"() -> (w469:refnum<vi>)
            n279 = call <userlib>:"Write Panel to INI__ogtk.vi"("error in (no error)"=w467, "VI ref"=w469, "refnum"=w470) -> ("error out"=w466:errorcluster, "refnum out"=w468:T18)  [unwired: 7 in]
            n280 = call <vilib>:"Close Config Data.vi"("error in (no error)"=w466, "refnum"=w468) -> ("error out"=w461:errorcluster, "file path"=w460:path)  [unwired: 8 in]
            n281 = Open/Create/Replace File(file path (use dialog)=w460, error in=w461) -> (refnum out=w464:refnum<file>, error out=w465:errorcluster)  [unwired: 4 in, 1 out]
            n282 = Flush File(refnum=w464, error in=w465) -> (refnum out=w463:refnum<file>, error out=w462:errorcluster)
            n283 = Close File(refnum=w463, error in=w462) -> ()  [unwired: 2 out]
          }
        }
      }
      event "手动启动": Value Change {
        n284 = event-data() -> ()  [unwired: 1 in, 6 out]
        n285 = call "氨氮启动参数对话框.vi"() -> ("确认"=w474:bool, "元素"=w475:cluster{"命令":string, "data":variant})  [unwired: 10 in]
        n286 = case shown="真" w474 {
          tunnel: w476 -> [_ w478]
          tunnel: w475 -> [_ w477]
          frame False {
          }
          frame True {
            n287 = Enqueue Element(queue=w478, element=w477) -> ()  [unwired: 2 in, 3 out]
          }
        }
      }
      event "定时启动": Mouse Down {
        n288 = event-data() -> ()  [unwired: 1 in, 6 out]
        n289 = flat-sequence {
          frame #0 {
            n290 = global read "氨氮断电保存全局变量.vi" "定时控制"() -> (w479:T7)
            n291 = call "周期设置.vi"("定时控制参数输入"=w479) -> ("定时控制参数输出"=w480:T7)  [unwired: 10 in]
            n292 = global write "氨氮断电保存全局变量.vi" "定时控制"(w480) -> ()
          }
          frame #1 {
            n293 = call <vilib>:"Application Directory.vi"() -> ("Application Directory"=w494:path)
            n294 = Build Path(base path=w494, name or relative path="data\\sys.ini" ("名称或相对路径")) -> (appended path=w492:path)
            n295 = call <vilib>:"Open Config Data.vi"("configuration file path"=w492) -> ("error out"=w488:errorcluster, "refnum"=w491:T18)  [unwired: 8 in, 1 out]
            n296 = vi-ref "氨氮断电保存全局变量.vi"() -> (w490:refnum<vi>)
            n297 = call <userlib>:"Write Panel to INI__ogtk.vi"("error in (no error)"=w488, "VI ref"=w490, "refnum"=w491) -> ("error out"=w487:errorcluster, "refnum out"=w489:T18)  [unwired: 7 in]
            n298 = call <vilib>:"Close Config Data.vi"("error in (no error)"=w487, "refnum"=w489) -> ("error out"=w482:errorcluster, "file path"=w481:path)  [unwired: 8 in]
            n299 = Open/Create/Replace File(file path (use dialog)=w481, error in=w482) -> (refnum out=w485:refnum<file>, error out=w486:errorcluster)  [unwired: 4 in, 1 out]
            n300 = Flush File(refnum=w485, error in=w486) -> (refnum out=w484:refnum<file>, error out=w483:errorcluster)
            n301 = Close File(refnum=w484, error in=w483) -> ()  [unwired: 2 out]
          }
        }
      }
      event "单步测试": Value Change {
        w496 = u16 1 items=["总磷"=1, "氨氮"=3] ("站号")
        n302 = event-data() -> ()  [unwired: 1 in, 6 out]
        n303 = Bundle("站号"=w496, "总磷氨氮调试"="总磷氨氮调试") -> (w495:cluster{"站号":u16, "总磷氨氮调试":u16[]})  [unwired: 1 in]
        n304 = Bundle By Name(cluster=cluster{"命令":string, "data":variant} {"命令"="", "data"=variant} ("元素"), "命令"="debug", "data"=w495) -> (w498:cluster{"命令":string, "data":variant})
        n305 = Enqueue Element(queue=w501, element=w498) -> ()  [unwired: 2 in, 3 out]
      }
      event "停止": Value Change {
        n306 = event-data() -> ()  [unwired: 1 in, 6 out]
        n307 = Enqueue Element(queue=w506, element=cluster{"命令":string, "data":variant} {"命令"="启动", "data"=variant(cluster{"站号":u16, "控制命令输出":u16[]} {"站号"=3, "控制命令输出"=[2816]})} ("启动命令")) -> ()  [unwired: 2 in, 3 out]
        n308 = Cancel Notification(0:w504) -> (8:w503:refnum<notifier>)  [unwired: 1 in, 2 out]
        n309 = Send Notification(notification=TRUE ("通知"), notifier=w503) -> ()  [unwired: 1 in, 2 out]
      }
      event "设置": Value Change {
        n310 = event-data() -> ()  [unwired: 1 in, 6 out]
        n311 = property on="窗格" class="Pane"("Origin"=T10 {"Horizontal"=0, "Vertical"=628} ("原点")) -> ()  [unwired: 2 in, 2 out]
      }
      event "返回": Value Change {
        n312 = event-data() -> ()  [unwired: 1 in, 6 out]
        n313 = property on="窗格" class="Pane"("Origin"=T10 {"Horizontal"=0, "Vertical"=0} ("原点")) -> ()  [unwired: 2 in, 2 out]
      }
      event "公式.X^2", "公式.X", "公式.b", "量程切换阈值.阈值", "量程切换阈值.标液浓度", "备用系数.量程上限", "备用系数.量程下限", "备用系数.检出限", "备用系数.精度": Mouse Down {
        n314 = event-data() -> ("CtlRef"=w512:refnum<vi>)  [unwired: 1 in, 5 out]
        n315 = property class="DigNum (严格)"(reference=w512) -> (reference out=w510:refnum<vi>, "Value"=w511:dbl)  [unwired: 1 in, 1 out]
        n316 = call "数字键盘.vi"("OldNumber"=w511) -> ("NewNumber"=w509:dbl)
        n317 = property class="DigNum (严格)"(reference=w510, "Val(Sgnl)"=w509) -> ()  [unwired: 1 in, 2 out]
      }
      event "读公式": Value Change {
        n318 = event-data() -> ()  [unwired: 1 in, 6 out]
        n319 = property class="Enum (严格)"(reference=w520) -> ("Value"=w519:enum16{"氨氮", "总磷"})  [unwired: 1 in, 2 out]
        n320 = property class="Enum (严格)"(reference=w521) -> ("Value"=w518:enum16{"水样测量", "空白核查", "跨度核查", "标样核查", "加标回收"})  [unwired: 1 in, 2 out]
        n321 = property class="Enum (严格)"(reference=w522) -> ("Value"=w517:enum16{"低量程", "高量程"})  [unwired: 1 in, 2 out]
        n322 = call "氨氮公式读取.vi"("量程"=w517, "测量模式"=w518, "测量参数"=w519) -> ("error out"=w514:errorcluster, "公式"=w515:cluster{"X^2":dbl, "X":dbl, "b":dbl})  [unwired: 7 in]
        n323 = property class="Clust (严格)"(reference=w516, "Value"=w515) -> ()  [unwired: 1 in, 2 out]
        n324 = case shown="错误" w514 {
          tunnel: ["读取成功" ("消息") "读取失败" ("消息")] -> w513
          frame No Error {
          }
          frame Error {
          }
        }
        n325 = One Button Dialog(message=w513) -> ()  [unwired: 1 in, 1 out]
      }
      event "写公式": Value Change {
        n326 = event-data() -> ()  [unwired: 1 in, 6 out]
        n327 = call "氨氮公式写入.vi"("公式"="公式", "量程"="量程下拉列表", "测量模式"="测量模式下拉列表", "测量参数"="参数下拉列表") -> ("error out"=w525:errorcluster)  [unwired: 7 in]
        n328 = case shown="无错误" w525 {
          tunnel: ["写入成功" ("消息") "写入失败" ("消息")] -> w526
          frame No Error {
          }
          frame Error {
          }
        }
        n329 = One Button Dialog(message=w526) -> ()  [unwired: 1 in, 1 out]
      }
      event "量程切换阈值读取": Value Change {
        n330 = event-data() -> ()  [unwired: 1 in, 6 out]
        n331 = property class="Enum (严格)"(reference=w540) -> ("Value"=w539:enum16{"氨氮", "总磷"})  [unwired: 1 in, 2 out]
        n332 = property class="Enum (严格)"(reference=w541) -> ("Value"=w538:enum16{"水样测量", "空白核查", "跨度核查", "标样核查", "加标回收"})  [unwired: 1 in, 2 out]
        n333 = property class="Enum (严格)"(reference=w542) -> ("Value"=w537:enum16{"低量程", "高量程"})  [unwired: 1 in, 2 out]
        n334 = call "氨氮量程读取.vi"("量程"=w537, "测量模式"=w538, "测量参数"=w539) -> ("error out"=w533:errorcluster, "量程切换阈值"=w535:cluster{"阈值":dbl, "标液浓度":dbl})  [unwired: 7 in]
        n335 = property class="Clust (严格)"(reference=w536, "Value"=w535) -> ()  [unwired: 1 in, 2 out]
        n336 = case shown="错误" w533 {
          tunnel: ["读取成功" ("消息") "读取失败" ("消息")] -> w534
          frame No Error {
          }
          frame Error {
          }
        }
        n337 = One Button Dialog(message=w534) -> ()  [unwired: 1 in, 1 out]
      }
      event "量程切换阈值写入": Value Change {
        n338 = event-data() -> ()  [unwired: 1 in, 6 out]
        n339 = property class="Enum (严格)"(reference=w553) -> ("Value"=w550:enum16{"氨氮", "总磷"})  [unwired: 1 in, 2 out]
        n340 = property class="Enum (严格)"(reference=w552) -> ("Value"=w549:enum16{"水样测量", "空白核查", "跨度核查", "标样核查", "加标回收"})  [unwired: 1 in, 2 out]
        n341 = property class="Enum (严格)"(reference=w551) -> ("Value"=w548:enum16{"低量程", "高量程"})  [unwired: 1 in, 2 out]
        n342 = call "氨氮量程写入.vi"("量程切换阈值"="量程切换阈值", "量程"=w548, "测量模式"=w549, "测量参数"=w550) -> ("error out"=w545:errorcluster)  [unwired: 7 in]
        n343 = case shown="无错误" w545 {
          tunnel: ["写入成功" ("消息") "写入失败" ("消息")] -> w546
          frame No Error {
          }
          frame Error {
          }
        }
        n344 = One Button Dialog(message=w546) -> ()  [unwired: 1 in, 1 out]
      }
      event "备用系数读取": Value Change {
        n345 = event-data() -> ()  [unwired: 1 in, 6 out]
        n346 = property class="Enum (严格)"(reference=w565) -> ("Value"=w564:enum16{"氨氮", "总磷"})  [unwired: 1 in, 2 out]
        n347 = property class="Enum (严格)"(reference=w559) -> ("Value"=w556:enum16{"水样测量", "空白核查", "跨度核查", "标样核查", "加标回收"})  [unwired: 1 in, 2 out]
        n348 = property class="Enum (严格)"(reference=w558) -> ("Value"=w557:enum16{"低量程", "高量程"})  [unwired: 1 in, 2 out]
        n349 = call "氨氮备用系数读取.vi"("量程"=w557, "测量模式"=w556, "测量参数"=w564) -> ("error out"=w560:errorcluster, "备用系数"=w562:T2)  [unwired: 7 in]
        n350 = property class="Clust (严格)"(reference=w563, "Value"=w562) -> ()  [unwired: 1 in, 2 out]
        n351 = case shown="错误" w560 {
          tunnel: ["读取成功" ("消息") "读取失败" ("消息")] -> w561
          frame No Error {
          }
          frame Error {
          }
        }
        n352 = One Button Dialog(message=w561) -> ()  [unwired: 1 in, 1 out]
      }
      event "备用系数写入": Value Change {
        n353 = event-data() -> ()  [unwired: 1 in, 6 out]
        n354 = property class="Enum (严格)"(reference=w576) -> ("Value"=w575:enum16{"氨氮", "总磷"})  [unwired: 1 in, 2 out]
        n355 = property class="Enum (严格)"(reference=w571) -> ("Value"=w570:enum16{"水样测量", "空白核查", "跨度核查", "标样核查", "加标回收"})  [unwired: 1 in, 2 out]
        n356 = property class="Enum (严格)"(reference=w569) -> ("Value"=w568:enum16{"低量程", "高量程"})  [unwired: 1 in, 2 out]
        n357 = call "氨氮备用系数写入.vi"("备用系数"="备用系数", "量程"=w568, "测量模式"=w570, "测量参数"=w575) -> ("error out"=w572:errorcluster)  [unwired: 7 in]
        n358 = case shown="无错误" w572 {
          tunnel: ["写入成功" ("消息") "写入失败" ("消息")] -> w573
          frame No Error {
          }
          frame Error {
          }
        }
        n359 = One Button Dialog(message=w573) -> ()  [unwired: 1 in, 1 out]
      }
    }
  }
